vi "create channels for tags.vi"(10 "tags in":T1[](array[typedef]), 11 "EIP Tags Configuration in":refnum<class "EIP Tags Configuration.lvclass">) -> (0 "error out":errorcluster, 2 "channels":refnum<class "EIP Tags Channel.lvclass">[](array[class]), 3 "EIP Tags Configuration out":refnum<class "EIP Tags Configuration.lvclass">)   [LabVIEW 2013, in "EIP Tags editor node.lvclass"]
uses:
  EIP Tags editor node.lvclass
  <vilib>/NI/TBM Modules/EIP Tags/channel/EIP Tags Channel.lvclass
  <vilib>/NI/TBM Modules/EIP Tags/configuration/eip tag definition.ctl
  <vilib>/NI/TBM Modules/EIP Tags/configuration/eip tag types.ctl
  <vilib>/NI/TBM Modules/EIP Tags/configuration/EIP Tags Configuration.lvclass
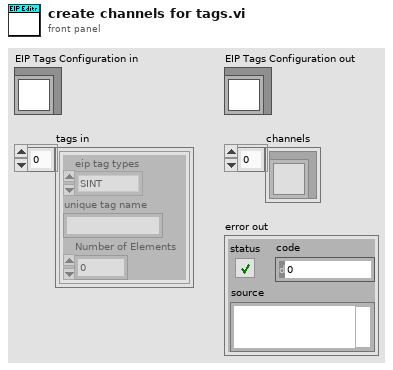
[diagram p1: front panel]
types:
  T1 = typedef "EIP Tags Configuration.lvclass/eip tag definition.ctl" = cluster{"eip tag types":T2, "unique tag name":string, "Number of Elements":u32}
  T2 = typedef "EIP Tags Configuration.lvclass/eip tag types.ctl" = enum16{"SINT", "INT", "DINT", "REAL", "BOOL", "STRING"}
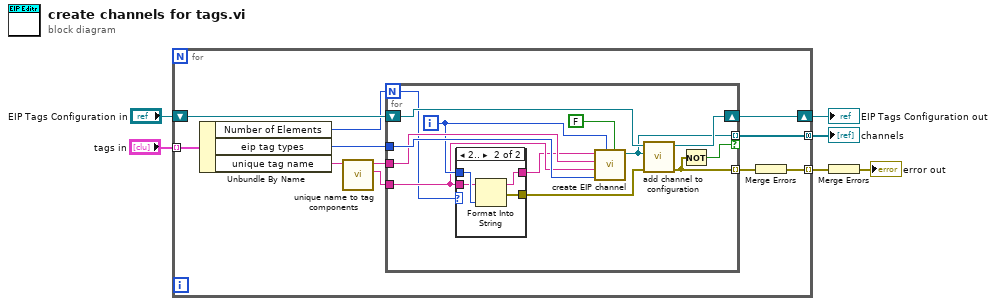
[diagram p0: block diagram]
diagram:
  n1 = for {
    shift-right: [w17] -> w4
    shift-left: "EIP Tags Configuration in" -> [w16]
    tunnel: [w15] -> w6 mode=concatenating
    tunnel: [w12] -> w2 mode=indexing
    tunnel: "tags in" -> [w13] mode=indexing
    n2 = Unbundle By Name(w13) -> ("Number of Elements"=w11:u32, "eip tag types"=w9:T2, "unique tag name"=w10:string)
    n3 = call <vilib>:"unique name to tag components.vi"("unique name"=w10) -> ("Tag Name"=w7:string, "Network Path"=w8:string)  [unwired: 9 in]
    n4 = for {
      N: w11 -> [w18]
      tunnel: [w28] -> w15 mode=indexing if=w26
      tunnel: [w27] -> w14 mode=indexing
      shift-right: [w30] -> w17
      shift-left: w16 -> [w29]
      tunnel: w9 -> [w25]
      tunnel: w8 -> [w24]
      tunnel: w7 -> [w22]
      i -> [w23]
      n5 = case shown="2.." w18 {
        tunnel: w23 -> [_ w35]
        tunnel: w22 -> [w31 w34]
        tunnel: [w31 w33] -> w21
        tunnel: [_ w32] -> w20
        frame ..1 {
        }
        frame 2.. {
          n6 = Format Into String(initial string=w34, w35) -> (resulting string=w33:string, error out=w32:errorcluster)  [unwired: 2 in]
        }
      }
      n7 = call <vilib>:"create EIP channel.vi"("output?"=FALSE, "element index"=w23, "eip tag type"=w25, "Tag Name"=w22, "Network Path"=w24, "name"=w21) -> ("EthernetIP Channel out"=w28:refnum<class "EIP Tags Channel.lvclass">)  [unwired: 5 in]
      n8 = call <vilib>:"add channel to configuration.vi"("error in"=w20, "TBM channel in"=w28, "EthernetIP configuration in"=w29) -> ("error out"=w27:errorcluster, "EthernetIP configuration out"=w30:refnum<class "EIP Tags Configuration.lvclass">)  [unwired: 7 in]
      n9 = Not(x=w27) -> (.not. x?=w26:bool)
    }
    n10 = Merge Errors(w14) -> (w12:errorcluster)
  }
  "channels" <- w6
  "EIP Tags Configuration out" <- w4
  n11 = Merge Errors(w2) -> (→"error out":errorcluster)
